vi "DataTreeCtrlFM stateMachine.vi"(6 "newRemark":string, 7 "Func":T1, 8 "error in (no error)":errorcluster, 9 "multiDatasName":string[](array[string]), 10 "singleDataName":string, 11 "tdmsFilePath in":path) -> (0 "error out":errorcluster, 1 "dataList":string[](array[string]), 2 "signalData":waveform(sgl), 3 "tdmsFilePath out":path, 4 "outputArr":string[][](array[string]), 5 "valid":bool)   [LabVIEW 2018, in "DataTreeCtrl.lvclass"]
uses:
  DataTreeCtrl.lvclass
  ctl/FMstateMachineEnum.ctl
  PublicSubVI/Class/FileManager/FM/ctl/_PC_Pub_FM fileReadFuncEnum.ctl
  <vilib>/Utility/error.llb/Error Cluster From Error Code.vi
  <vilib>/ErrorRing/Error Ring.xnode
  PublicSubVI/Class/FileManager/TDMSAdv.lvclass
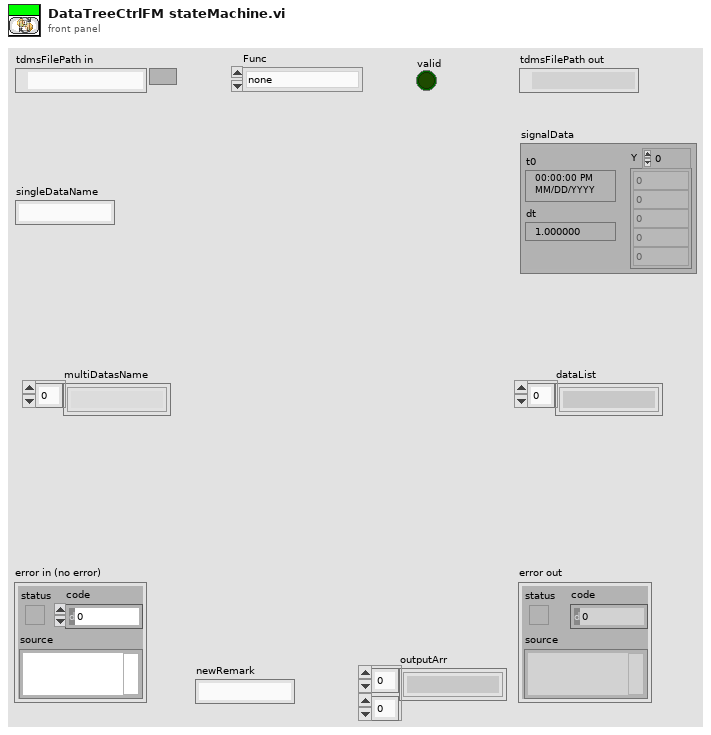
[diagram p1: front panel]
types:
  T1 = typedef "FMstateMachineEnum.ctl" = enum16{"none", "init", "openTDMS", "closeTDMS", "getDataList", "getDataInfo", "getTimeStamp", "getCurrPath", "getRemark", "overwriteRemark", "readData", "deleteData", "moveData"}
  T2 = enum16{"open", "open or create", "create or replace", "create", "open (read-only)"}
  T3 = typedef "_PC_Pub_FM fileReadFuncEnum.ctl" = enum16{"getAllInfo", "getChromatogram", "getDataItems", "getTimeStamp", "getIdxData", "getIonization", "getRemark", "getAttrFormat"}
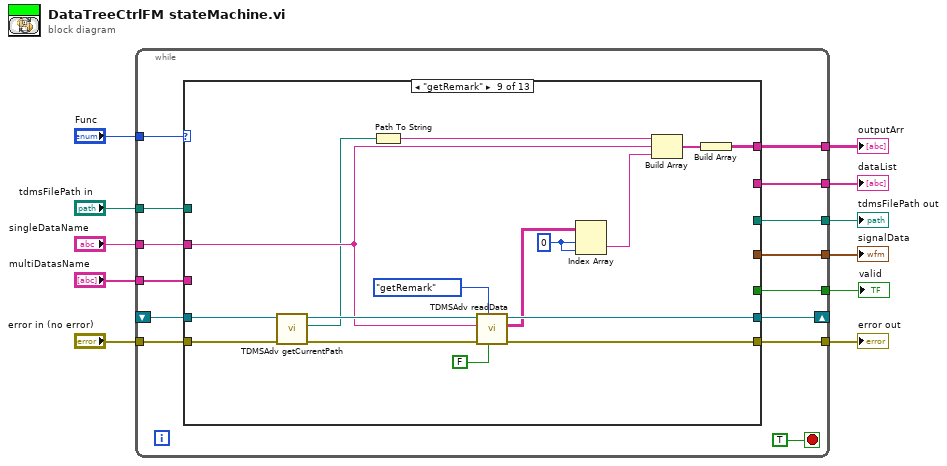
[diagram p0: block diagram]
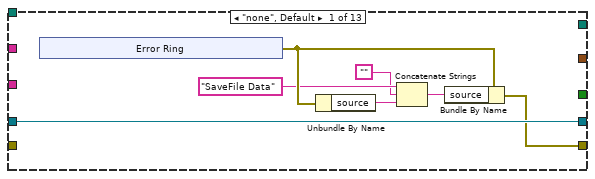
[diagram p2: hidden frame]
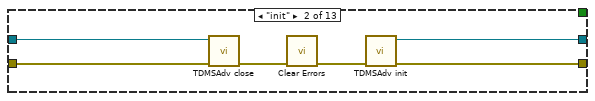
[diagram p3: hidden frame]
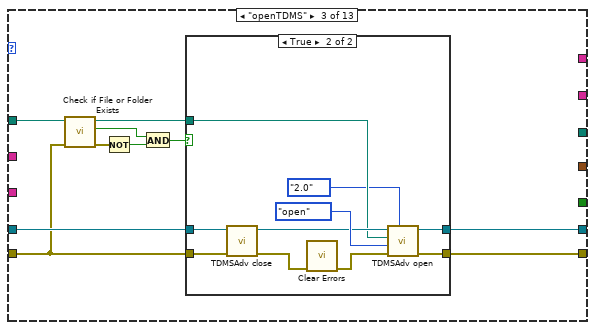
[diagram p4: hidden frame]
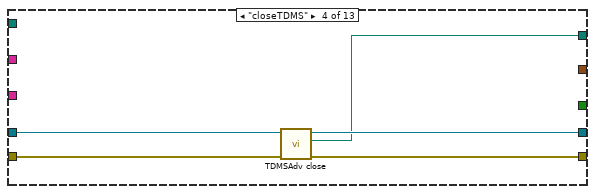
[diagram p6: hidden frame]
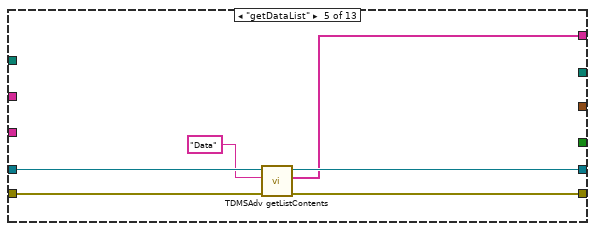
[diagram p7: hidden frame]
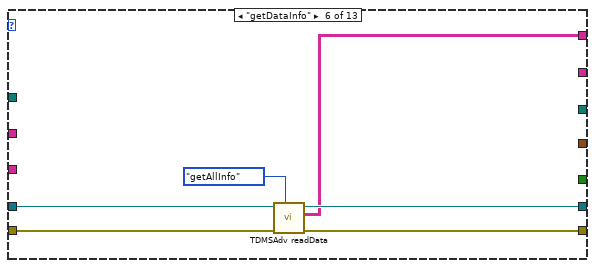
[diagram p8: hidden frame]
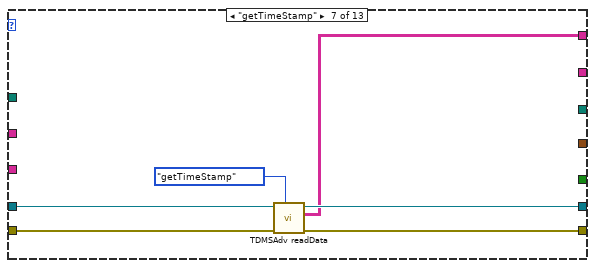
[diagram p9: hidden frame]
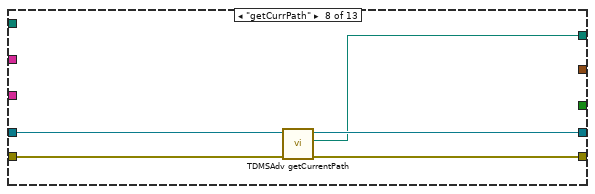
[diagram p10: hidden frame]
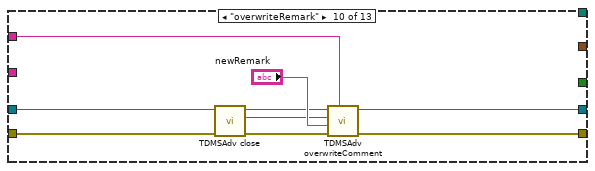
[diagram p11: hidden frame]
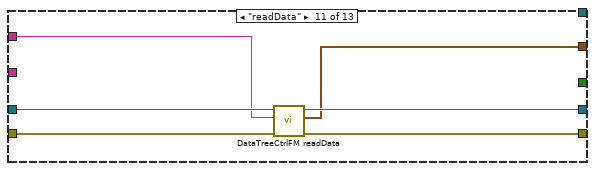
[diagram p12: hidden frame]
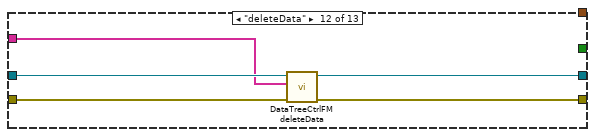
[diagram p13: hidden frame]
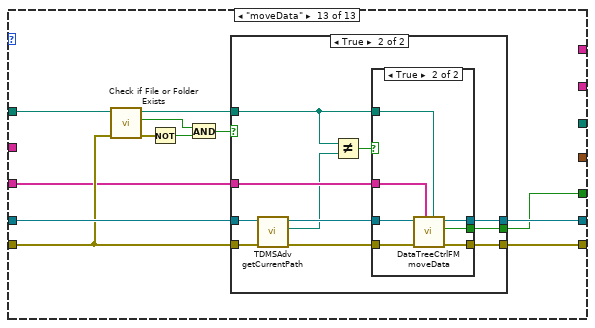
[diagram p14: hidden frame]
diagram:
  n1 = while {
    tunnel: "Func" -> [w25]
    shift-right: [w24] -> _
    shift-left: _ -> [w23]
    tunnel: "error in (no error)" -> [w22]
    tunnel: [w21] -> w9
    tunnel: "tdmsFilePath in" -> [w19]
    tunnel: [w18] -> w7
    tunnel: "multiDatasName" -> [w17]
    tunnel: [w16] -> w3
    tunnel: [w15] -> w6
    tunnel: [w14] -> w5
    tunnel: "singleDataName" -> [w13]
    tunnel: [w12] -> w1
    stop <- TRUE stop-if-true
    n2 = case shown="\"getRemark\"" w25 {
      tunnel: [w32 w42 w52 w68 w73 w77 w83 w91 w103 w112 w123 w125 w132] -> w24
      tunnel: w23 -> [w32 w40 w50 w69 w75 w81 w87 w92 w108 w116 w121 w128 w140]
      tunnel: w22 -> [_ w39 w46 w66 w74 w80 w86 w89 w107 w113 w120 w127 w135]
      tunnel: [w26 w41 w51 w67 w72 w78 w84 w90 w104 w109 w122 w124 w131] -> w21
      tunnel: w19 -> [_ _ w49 _ _ _ _ _ _ _ _ _ w136]
      tunnel: [_ _ _ w65 _ _ _ w88 _ _ _ _ _] -> w18
      tunnel: w17 -> [_ _ _ _ _ _ _ _ _ _ _ w126 w130]
      tunnel: [_ _ _ _ _ _ _ _ _ _ w119 _ _] -> w16
      tunnel: [_ _ _ _ w71 _ _ _ _ _ _ _ _] -> w15
      tunnel: [_ _ _ _ _ w76 w82 _ w97 _ _ _ _] -> w14
      tunnel: w13 -> [_ _ _ _ _ _ _ _ w96 w111 w118 _ _]
      tunnel: [_ _ _ _ _ _ _ _ _ _ _ _ w129] -> w12
      frame "none", Default {
        n3 = xnode "Error Ring"() -> ("error out"=w31:errorcluster)
        n4 = Unbundle By Name(w31) -> ("source"=w30:string)
        n5 = Concatenate Strings("SaveFile Data" ("string"), "", w30) -> (w29:string)
        n6 = Bundle By Name(cluster=w31, "source"=w29) -> (w26:errorcluster)
      }
      frame "init" {
        n7 = call "TDMSAdv close.vi"("error in (no error)"=w39, "TDMSAdv in"=w40) -> ("error out"=w38:errorcluster)  [unwired: 7 in, 2 out]
        n8 = call <vilib>:"Clear Errors.vi"("error in (no error)"=w38) -> ("error out"=w37:errorcluster)  [unwired: 5 in, 1 out]
        n9 = call "TDMSAdv init.vi"("error in (no error)"=w37) -> ("error out"=w41:errorcluster, "TDMSAdv out"=w42:refnum<class "TDMSAdv.lvclass">)  [unwired: 9 in]
      }
      frame "openTDMS" {
        n10 = call <vilib>:"Check if File or Folder Exists.vi"("error in (no error)"=w46, "path"=w49) -> ("error out"=w47:errorcluster, "file or folder exists?"=w45:bool, "dup path"=w48:path)  [unwired: 7 in]
        n11 = Not(x=w47) -> (.not. x?=w44:bool)
        n12 = And(x=w45, y=w44) -> (x .and. y?=w43:bool)
        n13 = case shown="True" w43 {
          tunnel: [w54 w63] -> w52
          tunnel: [w53 w62] -> w51
          tunnel: w50 -> [w54 w61]
          tunnel: w48 -> [_ w57]
          tunnel: w46 -> [w53 w56]
          frame False {
          }
          frame True {
            n14 = call "TDMSAdv close.vi"("error in (no error)"=w56, "TDMSAdv in"=w61) -> ("error out"=w59:errorcluster, "TDMSAdv out"=w60:refnum<class "TDMSAdv.lvclass">)  [unwired: 7 in, 1 out]
            n15 = call <vilib>:"Clear Errors.vi"("error in (no error)"=w59) -> ("error out"=w58:errorcluster)  [unwired: 5 in, 1 out]
            n16 = call "TDMSAdv open.vi"("file format version"=enum16{"1.0", "2.0", "Adv"}."2.0", "error in (no error)"=w58, "operation (0:open)"=T2."open", "openPath"=w57, "TDMSAdv in"=w60) -> ("error out"=w62:errorcluster, "TDMSAdv out"=w63:refnum<class "TDMSAdv.lvclass">)  [unwired: 5 in]
          }
        }
      }
      frame "closeTDMS" {
        n17 = call "TDMSAdv close.vi"("error in (no error)"=w66, "TDMSAdv in"=w69) -> ("error out"=w67:errorcluster, "filePath"=w65:path, "TDMSAdv out"=w68:refnum<class "TDMSAdv.lvclass">)  [unwired: 7 in]
      }
      frame "getDataList" {
        n18 = call "TDMSAdv getListContents.vi"("error in (no error)"=w74, "group name"="Data", "TDMSAdv in"=w75) -> ("error out"=w72:errorcluster, "channels"=w71:string[], "TDMSAdv out"=w73:refnum<class "TDMSAdv.lvclass">)  [unwired: 6 in]
      }
      frame "getDataInfo" {
        n19 = call "TDMSAdv readData.vi"("readEvent"=_PC_Pub_FM_fileReadFuncEnum."getAllInfo", "error in (no error)"=w80, "TDMSAdv in"=w81) -> ("error out"=w78:errorcluster, "outputArr"=w76:string[][], "TDMSAdv out"=w77:refnum<class "TDMSAdv.lvclass">)  [unwired: 5 in, 1 out]
      }
      frame "getTimeStamp" {
        n20 = call "TDMSAdv readData.vi"("readEvent"=_PC_Pub_FM_fileReadFuncEnum."getTimeStamp", "error in (no error)"=w86, "TDMSAdv in"=w87) -> ("error out"=w84:errorcluster, "outputArr"=w82:string[][], "TDMSAdv out"=w83:refnum<class "TDMSAdv.lvclass">)  [unwired: 5 in, 1 out]
      }
      frame "getCurrPath" {
        n21 = call "TDMSAdv getCurrentPath.vi"("error in (no error)"=w89, "TDMSAdv in"=w92) -> ("error out"=w90:errorcluster, "currFIlePath"=w88:path, "TDMSAdv out"=w91:refnum<class "TDMSAdv.lvclass">)  [unwired: 7 in]
      }
      frame "getRemark" {
        w100 = 0 ("index (row)")
        n22 = call "TDMSAdv getCurrentPath.vi"("error in (no error)"=w107, "TDMSAdv in"=w108) -> ("error out"=w105:errorcluster, "currFIlePath"=w94:path, "TDMSAdv out"=w106:refnum<class "TDMSAdv.lvclass">)  [unwired: 7 in]
        n23 = Path To String(path=w94) -> (string=w102:string)
        n24 = call "TDMSAdv readData.vi"("stringSplit? (T)"=FALSE, "readEvent"=_PC_Pub_FM_fileReadFuncEnum."getRemark", "error in (no error)"=w105, "timeStamp"=w96, "TDMSAdv in"=w106) -> ("error out"=w104:errorcluster, "outputArr"=w101:string[][], "TDMSAdv out"=w103:refnum<class "TDMSAdv.lvclass">)  [unwired: 3 in, 1 out]
        n25 = Index Array(array=w101, index (row)=w100, index (col)=w100) -> (element=w99:string)
        n26 = Build Array(w102, w96, w99) -> (w98:string[])
        n27 = Build Array(w98) -> (w97:string[][])
      }
      frame "overwriteRemark" {
        n28 = call "TDMSAdv close.vi"("error in (no error)"=w113, "TDMSAdv in"=w116) -> ("error out"=w114:errorcluster, "filePath"=w110:path, "TDMSAdv out"=w115:refnum<class "TDMSAdv.lvclass">)  [unwired: 7 in]
        n29 = call "TDMSAdv overwriteComment.vi"("timeStamp"=w111, "error in (no error)"=w114, "newComment"="newRemark", "file path"=w110, "TDMSAdv in"=w115) -> ("error out"=w109:errorcluster, "TDMSAdv out"=w112:refnum<class "TDMSAdv.lvclass">)  [unwired: 5 in]
      }
      frame "readData" {
        n30 = call "DataTreeCtrlFM readData.vi"("error in (no error)"=w120, "dataName"=w118, "TDMSAdv in"=w121) -> ("error out"=w122:errorcluster, "signalData"=w119:waveform(sgl), "TDMSAdv out"=w123:refnum<class "TDMSAdv.lvclass">)  [unwired: 6 in]
      }
      frame "deleteData" {
        n31 = call "DataTreeCtrlFM deleteData.vi"("error in (no error)"=w127, "deleteNames"=w126, "TDMSAdv in"=w128) -> ("error out"=w124:errorcluster, "TDMSAdv out"=w125:refnum<class "TDMSAdv.lvclass">)  [unwired: 7 in]
      }
      frame "moveData" {
        n32 = call <vilib>:"Check if File or Folder Exists.vi"("error in (no error)"=w135, "path"=w136) -> ("error out"=w139:errorcluster, "file or folder exists?"=w138:bool, "dup path"=w133:path)  [unwired: 7 in]
        n33 = Not(x=w139) -> (.not. x?=w137:bool)
        n34 = And(x=w138, y=w137) -> (x .and. y?=w134:bool)
        n35 = case shown="True" w134 {
          tunnel: w140 -> [w142 w153]
          tunnel: w135 -> [w141 w152]
          tunnel: w133 -> [_ w145]
          tunnel: [w142 w150] -> w132
          tunnel: [w141 w148] -> w131
          tunnel: w130 -> [_ w146]
          tunnel: [_ w143] -> w129
          frame False {
          }
          frame True {
            n36 = call "TDMSAdv getCurrentPath.vi"("error in (no error)"=w152, "TDMSAdv in"=w153) -> ("error out"=w147:errorcluster, "currFIlePath"=w144:path, "TDMSAdv out"=w149:refnum<class "TDMSAdv.lvclass">)  [unwired: 7 in]
            n37 = Not Equal?(x=w145, y=w144) -> (x != y?=w151:bool)
            n38 = case shown="True" w151 {
              tunnel: [w155 w160] -> w150
              tunnel: w149 -> [w155 w162]
              tunnel: [w154 w159] -> w148
              tunnel: w147 -> [w154 w161]
              tunnel: w146 -> [_ w157]
              tunnel: w145 -> [_ w158]
              tunnel: [_ w156] -> w143
              frame False {
              }
              frame True {
                n39 = call "DataTreeCtrlFM moveData.vi"("movePath"=w158, "moveNames"=w157, "error in (no error)"=w161, "TDMSAdv Class in"=w162) -> ("error out"=w159:errorcluster, "valid"=w156:bool, "TDMSAdv Class out"=w160:refnum<class "TDMSAdv.lvclass">)  [unwired: 5 in]
              }
            }
          }
        }
      }
    }
  }
  "error out" <- w9
  "tdmsFilePath out" <- w7
  "dataList" <- w6
  "outputArr" <- w5
  "signalData" <- w3
  "valid" <- w1
